vi "Conversion Lookup Table Initialize.vi"(8 "error in (no error)":errorcluster, 11 "J1939 Process Parameters":T2={"J1939 XNET Settings"={"XNET Database"="", "XNET Cluster"="", "CAN Port"="", "Baud rate [Bd]"=0, "Termination"=0, "Incoming Rate"=0, "Outcoming Rate"=1, "Write Decimation"=1}, "Incoming Single Point Configuraiton"={"Incoming Single Point Frame"={"ID"=[], "Conversion"=[], "Channel Array Positions"=[], "Frame Length"=[]}, "Channel Pairs"={"Chan Refs"=[], "Previous Chan Values"=[]}, "Read FIFO"=refnum}, "Outgoing Cyclic Configuraiton"={"Outgoing Cyclic Frame"={"ID"=[], "Conversion"=[], "Channel Array Positions"=[], "Frame Length"=[], "Transmit Propreties"=[]}, "Channel Pairs"={"Block Data Refs"=[], "Previous Chan Values"=[]}, "Write FIFO"=refnum}, "J1939 Monitor Settings"={"J1939 Network Address"=0, "Name"=0}, "Simulated Addresses"=[], "Simulated Addresses LUT"=variant, "Name"=""} {"Simulated Addresses"."Simulated Addresses"."J1939 XNET Settings"."Name" format="%.0x"; "Simulated Addresses"."Simulated Addresses"."DM1 Data"."Data Reference" format="%.0x"; "Simulated Addresses"."Simulated Addresses"."DM1 Enable?"."Data Reference" format="%.0x"; "Simulated Addresses"."Simulated Addresses"."DM2 Data"."Data Reference" format="%.0x"; "Simulated Addresses"."Simulated Addresses"."DM2 Enable?"."Data Reference" format="%.0x"; "J1939 Monitor Settings"."Name" format="%.0x"; "Outgoing Cyclic Configuraiton"."Channel Pairs"."Block Data Refs"."Data Reference" format="%.0x"; "Outgoing Cyclic Configuraiton"."Outgoing Cyclic Frame"."Transmit Propreties"."Transmit Time" format="%#_p"; "J1939 XNET Settings"."Termination" items=["Off", "On"]; "Incoming Single Point Configuraiton"."Channel Pairs"."Chan Refs" format="%.0x"}) -> (0 "error out":errorcluster {"code" min=0 max=0}, 3 "Scale Ref out":T1)   [LabVIEW 2015, in "J1939 Addon Engine.lvlib"]
uses:
  J1939 Addon Engine.lvlib
  Types/Process Parameters.ctl
  Shared/Types/XNET Settings.ctl
  Types/Incoming Single Point Configuration.ctl
  Types/Incoming Single Point Frame Pairs.ctl
  Shared/Types/Incoming Single Point Channel Pairs.ctl
  <vilib>/NI Veristand/Custom Device API/Data Reference.ctl
  Types/Outgoing Cyclic Configuration.ctl
  Types/Outgoing Cyclic Frame Pairs.ctl
  Shared/Types/XNET Frame Event Properties.ctl
  Shared/Types/Outgoing Cyclic Channel Pairs.ctl
  <vilib>/NI Veristand/Custom Device API/Block Data Reference.ctl
  Shared/Types/Monitor Settings.ctl
  Types/Simulated Settings.ctl
  Shared/Types/Compiled Simulated Settings.ctl
  Types/DTC FIFOs.ctl
  Types/Conversion Lookup Table Reference.ctl
  <vilib>/NI VeriStand/Custom Device API/Custom Device API.lvlib
  Shared/J1939 Addon Shared.lvlib
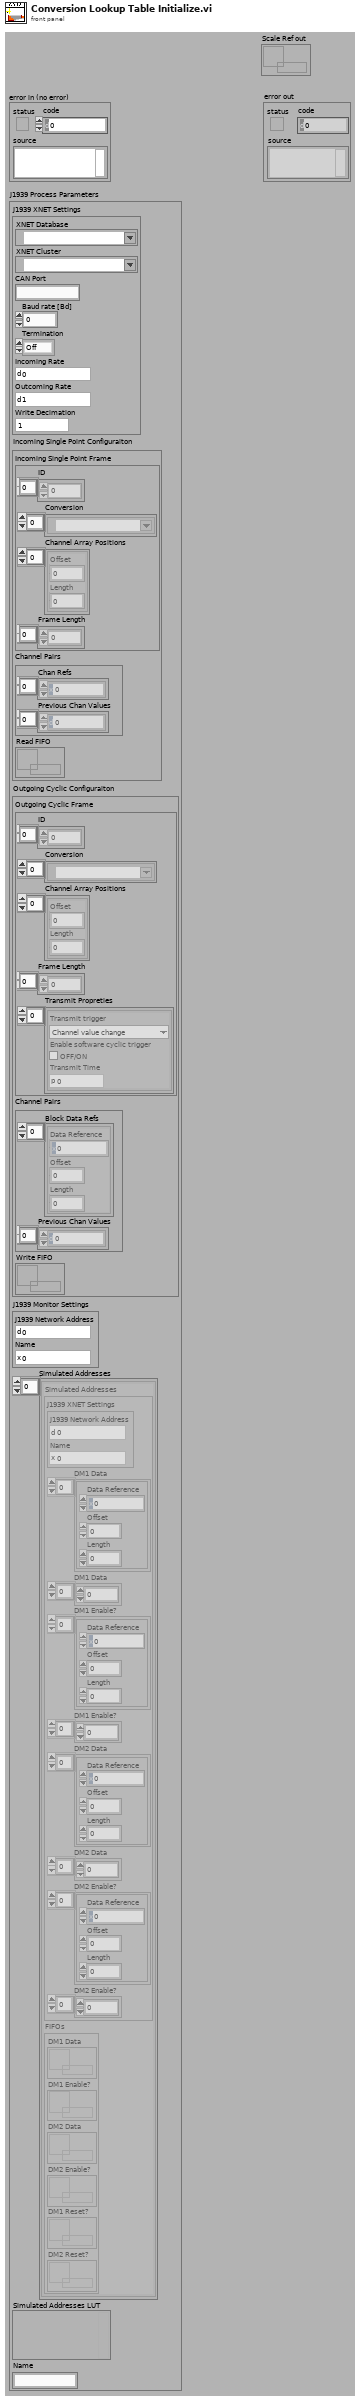
[diagram p1: front panel]
types:
  T1 = typedef "J1939 Addon Engine.lvlib/Conversion Lookup Table Reference.ctl" = refnum<data-value>
  T2 = typedef "J1939 Addon Engine.lvlib/Process Parameters.ctl" = cluster{"J1939 XNET Settings":T3, "Incoming Single Point Configuraiton":T4, "Outgoing Cyclic Configuraiton":T8, "J1939 Monitor Settings":T13, "Simulated Addresses":T14[], "Simulated Addresses LUT":variant, "Name":string}
  T3 = typedef "J1939 Addon Shared.lvlib/XNET Settings.ctl" = cluster{"XNET Database":refnum<k21>, "XNET Cluster":refnum<k21>, "CAN Port":string, "Baud rate [Bd]":u32, "Termination":u32, "Incoming Rate":u32, "Outcoming Rate":u32, "Write Decimation":u32}
  T4 = typedef "J1939 Addon Engine.lvlib/Incoming Single Point Configuration.ctl" = cluster{"Incoming Single Point Frame":T5, "Channel Pairs":T6, "Read FIFO":refnum<k33>}
  T5 = typedef "J1939 Addon Engine.lvlib/Incoming Single Point Frame Pairs.ctl" = cluster{"ID":u32[], "Conversion":refnum<k21>[], "Channel Array Positions":cluster{"Offset":u32, "Length":u32}[], "Frame Length":u32[]}
  T6 = typedef "J1939 Addon Shared.lvlib/Incoming Single Point Channel Pairs.ctl" = cluster{"Chan Refs":T7[], "Previous Chan Values":dbl[]}
  T7 = typedef "Custom Device API.lvlib/Data Reference.ctl" = i32
  T8 = typedef "J1939 Addon Engine.lvlib/Outgoing Cyclic Configuration.ctl" = cluster{"Outgoing Cyclic Frame":T9, "Channel Pairs":T11, "Write FIFO":refnum<k33>}
  T9 = typedef "J1939 Addon Engine.lvlib/Outgoing Cyclic Frame Pairs.ctl" = cluster{"ID":u32[], "Conversion":refnum<k21>[], "Channel Array Positions":cluster{"Offset":u32, "Length":u32}[], "Frame Length":u32[], "Transmit Propreties":T10[]}
  T10 = typedef "J1939 Addon Shared.lvlib/XNET Frame Event Properties.ctl" = cluster{"Transmit trigger":enum16{"Channel value change"}, "Enable software cyclic trigger":bool, "Transmit Time":dbl}
  T11 = typedef "J1939 Addon Shared.lvlib/Outgoing Cyclic Channel Pairs.ctl" = cluster{"Block Data Refs":T12[], "Previous Chan Values":dbl[]}
  T12 = typedef "Custom Device API.lvlib/Block Data Reference.ctl" = cluster{"Data Reference":T7, "Offset":u64, "Length":u64}
  T13 = typedef "J1939 Addon Shared.lvlib/Monitor Settings.ctl" = cluster{"J1939 Network Address":u8, "Name":u64}
  T14 = typedef "J1939 Addon Engine.lvlib/Simulated Settings.ctl" = cluster{"Simulated Addresses":T15, "FIFOs":T16}
  T15 = typedef "J1939 Addon Shared.lvlib/Compiled Simulated Settings.ctl" = cluster{"J1939 XNET Settings":T13, "DM1 Data":T12[], "DM1 Data":dbl[], "DM1 Enable?":T12[], "DM1 Enable?":dbl[], "DM2 Data":T12[], "DM2 Data":dbl[], "DM2 Enable?":T12[], "DM2 Enable?":dbl[]}
  T16 = typedef "J1939 Addon Engine.lvlib/DTC FIFOs.ctl" = cluster{"DM1 Data":refnum<k33>, "DM1 Enable?":refnum<k33>, "DM2 Data":refnum<k33>, "DM2 Enable?":refnum<k33>, "DM1 Reset?":refnum<k33>, "DM2 Reset?":refnum<k33>}
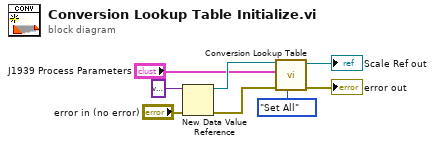
[diagram p0: block diagram]
diagram:
  n1 = New Data Value Reference(data value=variant ("variant"), error in="error in (no error)") -> (data value reference=w6:refnum<data-value>, error out=w5:errorcluster)
  n2 = call "Conversion Lookup Table.vi"("command"=enum16{"Set All", "Lookup Parameters"}."Set All", "error in (no error)"=w5, "J1939 Process Parameters"="J1939 Process Parameters", "Scale Ref"=w6) -> ("error out"=→"error out":errorcluster, "Scale Ref out"=→"Scale Ref out":T1)  [unwired: 4 in, 2 out]
